vi "Device Discovery Init.vi"(8 "error in":errorcluster, 11 "SCADA in":refnum<class "EMS.lvclass">) -> (0 "error out":errorcluster, 3 "SCADA out":refnum<class "EMS.lvclass">)   [LabVIEW 2018, in "EMS Core.lvlib" / "EMS.lvclass"]
uses:
  EMS.lvclass
  C:/Program Files (x86)/National Instruments/LabVIEW 2018/vi.lib/ActorFramework/Actor/Actor.lvclass
  Controls/Microgrid State.ctl
  EMS.lvclass/EMS.ctl
  <vilib>/ActorFramework/Actor/Actor.lvclass/Actor.ctl
  EMS Messages/Return Microgrid State Msg/Return Microgrid State Msg.lvclass/Return Microgrid State Msg.ctl
  <vilib>/ActorFramework/Message Enqueuer/Message Enqueuer.lvclass/Message Enqueuer.ctl
  <vilib>/ActorFramework/Message Enqueuer/Enqueue.vi
  EMS Messages/Return Microgrid State Msg/Return Microgrid State Msg.lvclass
  C:/Program Files (x86)/National Instruments/LabVIEW 2018/vi.lib/ActorFramework/Message/Message.lvclass
  <vilib>/ActorFramework/Message Priority Queue/Priority Enqueue.vi
  <vilib>/ActorFramework/Actor/Actor.lvclass
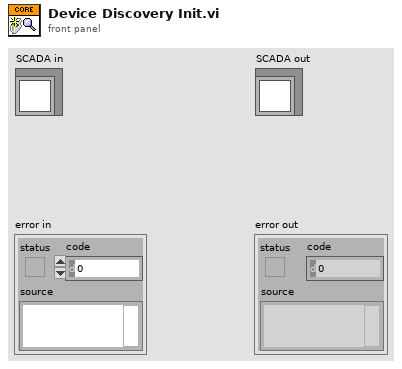
[diagram p1: front panel]
types:
  T1 = typedef "EMS Core.lvlib/EMS.lvclass/Microgrid State.ctl" = enum16{"Discovery", "Commissioning", "Activation", "Blackstart", "OnGrid", "OffGrid", "Island", "Resynchronization", "Manual", "Shutdown", "Stop"}
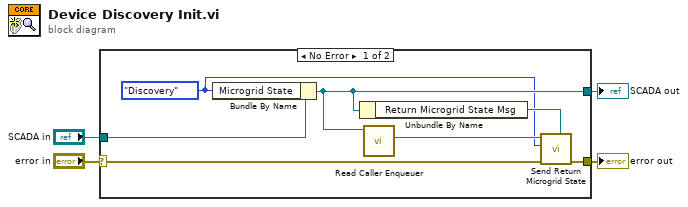
[diagram p0: block diagram]
diagram:
  n1 = case shown="No Error" "error in" {
    selector: "error in" -> [w10 w13]
    tunnel: [w7 w13] -> w3
    tunnel: [w6 w12] -> w1
    tunnel: "SCADA in" -> [w11 w12]
    frame No Error {
      w5 = Microgrid_State."Discovery" ("Microgrid State")
      n2 = Bundle By Name(cluster=w11, "Microgrid State"=w5) -> (w6:refnum<class "EMS.lvclass">)
      n3 = Unbundle By Name(w6) -> ("Return Microgrid State Msg"=w8:refnum<class "Return Microgrid State Msg.lvclass">)
      n4 = call <vilib>:"Read Caller Enqueuer.vi"("Actor"=w6) -> ("Caller Enqueuer"=w9:refnum<class "Message Enqueuer.lvclass">)  [unwired: 10 in]
      n5 = call "Send Return Microgrid State.vi"("Message Type"=w8, "error in (no error)"=w10, "Microgrid State"=w5, "Message Enqueuer"=w9) -> ("error out"=w7:errorcluster)  [unwired: 6 in, 1 out]
    }
    frame Error {
    }
  }
  "error out" <- w3
  "SCADA out" <- w1
